vi "Make VISA Name.vi"(1 "Instrument Address":refnum<visa-resource-name>) -> (0 "Name":string)   [LabVIEW 2020]
doc: "Makes a unique name from the VISA address. This is much more friendly to humans. It does not handle multiple GPIB buses.\nScott Hannahs, <sth@magnet.fsu.edu> NHMFL-FSU, May 2003"
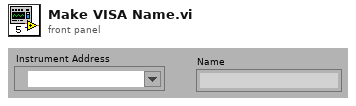
[diagram p1: front panel]
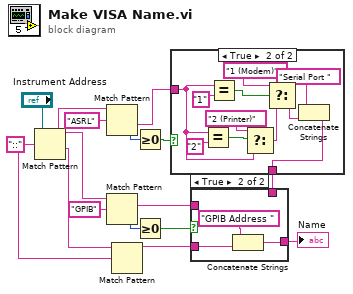
[diagram p0: block diagram]
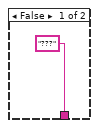
[diagram p3: hidden frame]
diagram:
  w15 = "::" ("regular expression")
  n1 = Match Pattern(string="Instrument Address", regular expression=w15) -> (before substring=w14:string, after substring=w4:string)  [unwired: 1 in, 2 out]
  n2 = Match Pattern(string=w14, regular expression="ASRL") -> (after substring=w10:string, offset past match=w11:i32)  [unwired: 1 in, 2 out]
  n3 = Match Pattern(string=w14, regular expression="GPIB") -> (match substring=w6:string, offset past match=w9:i32)  [unwired: 1 in, 2 out]
  n4 = Match Pattern(string=w4, regular expression=w15) -> (before substring=w5:string)  [unwired: 1 in, 3 out]
  n5 = Greater Or Equal To 0?(x=w11) -> (x >= 0?=w12:bool)
  n6 = Greater Or Equal To 0?(x=w9) -> (x >= 0?=w7:bool)
  n7 = case shown="True" w12 {
    tunnel: w10 -> [_ w18]
    tunnel: ["???" w23] -> w3
    frame False {
    }
    frame True {
      n8 = Equal?(x=w18, y="2") -> (x = y?=w20:bool)
      n9 = Equal?(x=w18, y="1") -> (x = y?=w27:bool)
      n10 = Select(t="2 (Printer)", s=w20, f=w18) -> (s? t:f=w17:string)
      n11 = Select(t="1 (Modem)", s=w27, f=w17) -> (s? t:f=w25:string)
      n12 = Concatenate Strings("Serial Port ", w25) -> (w23:string)
    }
  }
  n13 = case shown="True" w7 {
    tunnel: w6 -> [_ _]
    tunnel: w5 -> [_ w30]
    tunnel: w3 -> [w28 _]
    tunnel: [w28 w29] -> w2
    frame False {
    }
    frame True {
      n14 = Concatenate Strings("GPIB Address ", w30) -> (w29:string)
    }
  }
  "Name" <- w2
